vi "Font.vi"(11 "font":T1={"Name"="Arial", "Size"=16.0, "style"=0, "Color"={"Color"=0, "alpha"=76}} {"Color"."alpha" scale=0.0..255.0; "style" items=["Regular"=0, "Bold"=1, "Italic"=2, "Underline"=4, "Strikeout"=8]; "Size" min=4.0 max=100.0}) -> (3 ".NET MSChart Font":refnum<k24>)   [LabVIEW 2014, in "XMSChart.xctl"]
uses:
  XMSChart.xctl
  Controls/Font.ctl
  Controls/Color.ctl
  System.Drawing
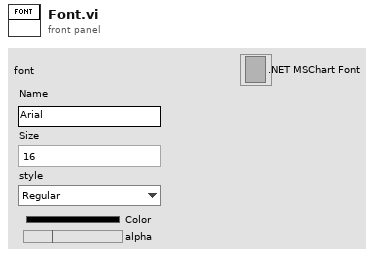
[diagram p1: front panel]
types:
  T1 = typedef "XMSChart.xctl/Font.ctl" = cluster{"Name":string, "Size":dbl, "style":i32, "Color":T2}
  T2 = typedef "XMSChart.xctl/Color.ctl" = cluster{"Color":u32, "alpha":u8}
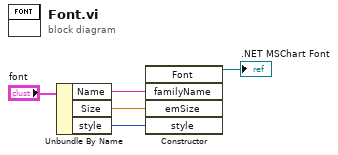
[diagram p0: block diagram]
diagram:
  n1 = Unbundle By Name("font") -> ("Name"=w4:string, "Size"=w3:dbl, "style"=w2:i32)
  n2 = constructor class="Font"("familyName"=w4, "emSize"=w3, "style"=w2) -> (reference out=→".NET MSChart Font":refnum<k24>)  [unwired: 3 in, 5 out]
